vi "RS232 S&R 3.vi"(4 "ReSetSPD":bool, 5 "error in":errorcluster, 6 "Delay (ms)":u32, 7 "Stage Control":T1={"Task"=0, "Position to go"={"Position"={"X"=FALSE, "Target X (um)"=1000.0, "Current X (um)"=1000.0, "Scaling X"=0, "Y"=FALSE, "Target Y (um)"=0.0, "Current Y (um)"=0.0, "Scaling Y"=0, "Z"=FALSE, "Target Z (um)"=0.0, "Current Z (um)"=0.0, "Scaling Z"=0}, "Speed"={"Speed"=3111, "Vi steps"=800, "Vi"=1000}}} {"Task" items=["MOVE", "HOME", "STOP", "Set Speed", "Info", "Set Zero", "MOVE2"]; "Position to go"."Speed"."Speed" min=50 max=8000 step=50 scale=50.0..8000.0; "Position to go"."Position"."Current X (um)" step=1.0; "Position to go"."Position"."Scaling Z" items=["X", "Z", "None"]; "Position to go"."Position"."Scaling Y" items=["X", "Z", "None"]; "Position to go"."Position"."Scaling X" items=["X", "Z", "None"]; "Position to go"."Position"."Target X (um)" step=1.0}, 8 "VISA resource in":refnum<visa-resource-name>) -> (0 "error out":errorcluster, 1 "read":bool, 2 "Cluster":T2={"Current coordinates"={"Steps"=0.0, "X"=FALSE, "Steps 2"=0.0, "Y"=FALSE, "Steps 3"=0.0, "Z"=FALSE}, "read buffer"="X0,Y0,Z0\r\n", "Command"="a", "Current coordinates 2"={"X"=0.0, "Y"=0.0, "Z"=0.0}, "Moving Time (Sec)"=0.0}, 3 "VISA resource name out":refnum<visa-resource-name>)   [LabVIEW 2018]
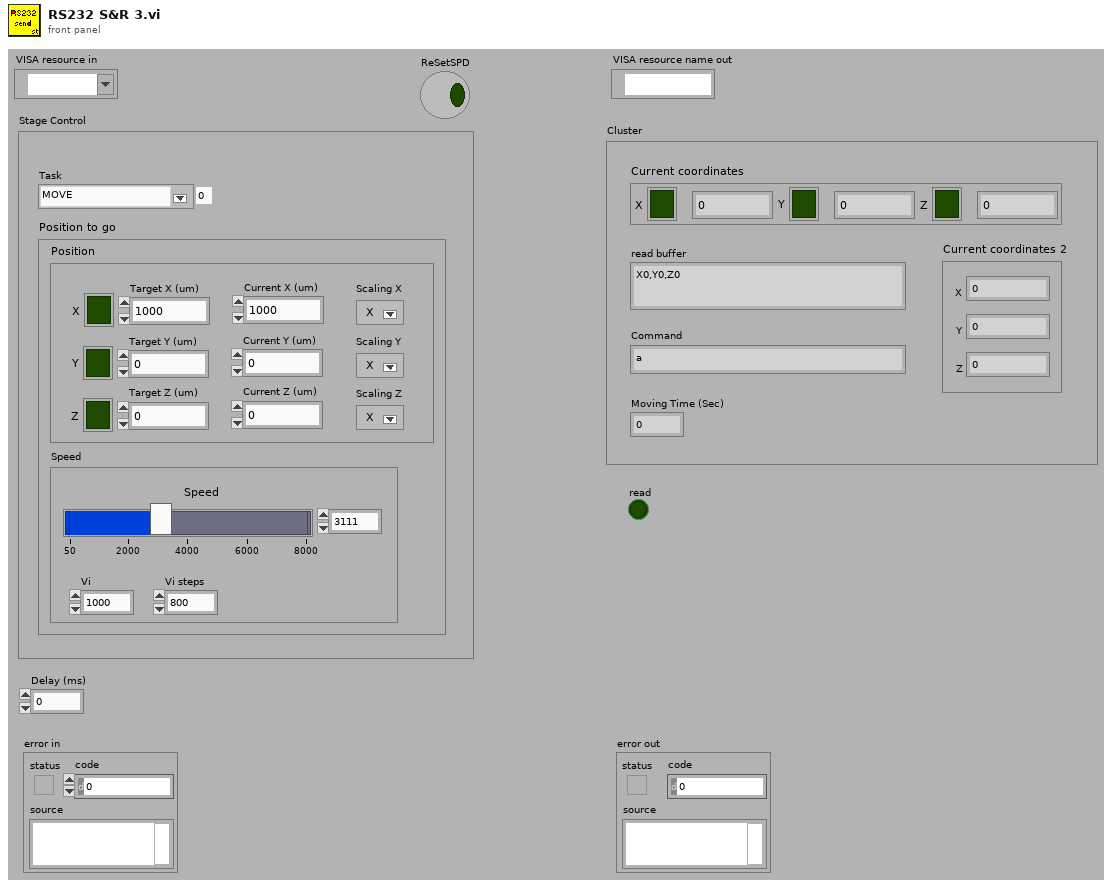
[diagram p1: front panel]
types:
  T1 = cluster{"Task":u16, "Position to go":cluster{"Position":cluster{"X":bool, "Target X (um)":dbl, "Current X (um)":dbl, "Scaling X":u16, "Y":bool, "Target Y (um)":dbl, "Current Y (um)":dbl, "Scaling Y":u16, "Z":bool, "Target Z (um)":dbl, "Current Z (um)":dbl, "Scaling Z":u16}, "Speed":cluster{"Speed":i32, "Vi steps":i32, "Vi":i32}}}
  T2 = cluster{"Current coordinates":cluster{"Steps":dbl, "X":bool, "Steps 2":dbl, "Y":bool, "Steps 3":dbl, "Z":bool}, "read buffer":string, "Command":string, "Current coordinates 2":cluster{"X":dbl, "Y":dbl, "Z":dbl}, "Moving Time (Sec)":dbl}
  T3 = cluster{"Position":cluster{"X":bool, "Target X (um)":dbl, "Current X (um)":dbl, "Scaling X":u16, "Y":bool, "Target Y (um)":dbl, "Current Y (um)":dbl, "Scaling Y":u16, "Z":bool, "Target Z (um)":dbl, "Current Z (um)":dbl, "Scaling Z":u16}, "Speed":cluster{"Speed":i32, "Vi steps":i32, "Vi":i32}}
  T4 = cluster{"X":bool, "Target X (um)":dbl, "Current X (um)":dbl, "Scaling X":u16, "Y":bool, "Target Y (um)":dbl, "Current Y (um)":dbl, "Scaling Y":u16, "Z":bool, "Target Z (um)":dbl, "Current Z (um)":dbl, "Scaling Z":u16}
  T5 = cluster{"X":bool, "Target X ":dbl, "Current X":dbl, "Scaling X":u16, "Y":bool, "Target Y":dbl, "Current Y":dbl, "Scaling Y":u16, "Z":bool, "Target Z":dbl, "Current Z":dbl, "Scaling Z":u16}
  T6 = cluster{"Steps":dbl, "X":bool, "Steps 2":dbl, "Y":bool, "Steps 3":dbl, "Z":bool}
  T7 = cluster{"Current coordinates":cluster{"Steps":dbl, "X":bool, "Steps 2":dbl, "Y":bool, "Steps 3":dbl, "Z":bool}, "read buffer":string, "command":string, cluster{"X":dbl, "Y":dbl, "Z":dbl}, dbl}
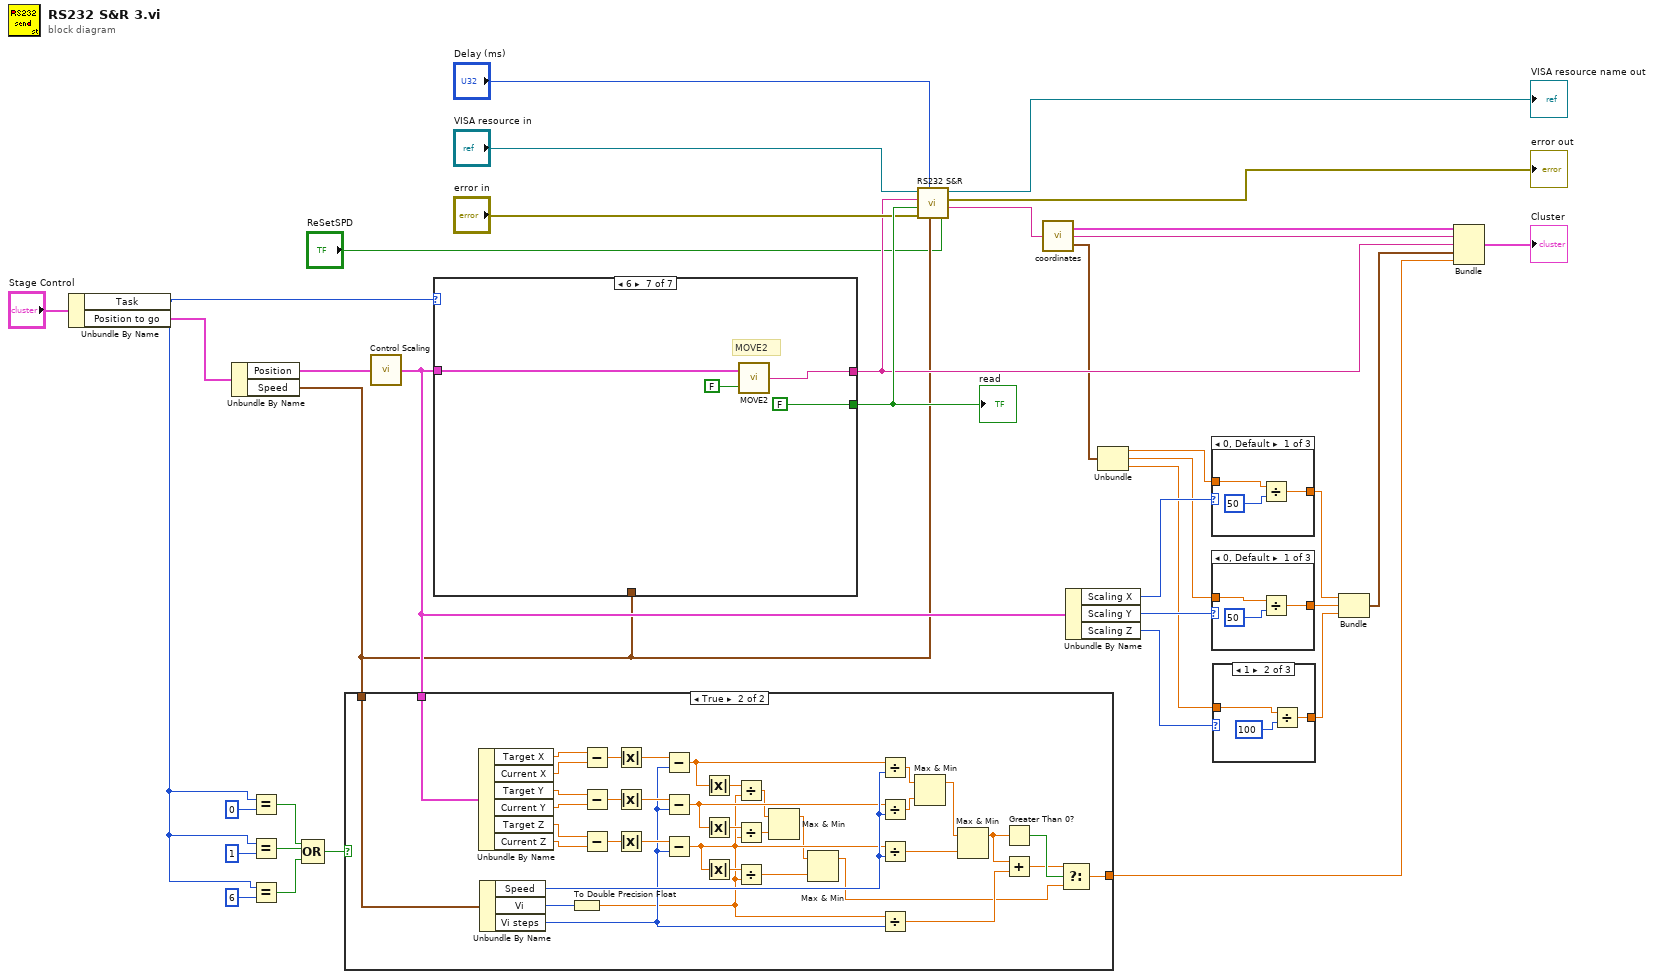
[diagram p0: block diagram]
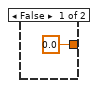
[diagram p2: hidden frame]
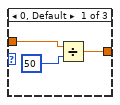
[diagram p3: hidden frame]
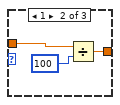
[diagram p5: hidden frame]
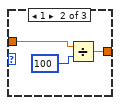
[diagram p7: hidden frame]
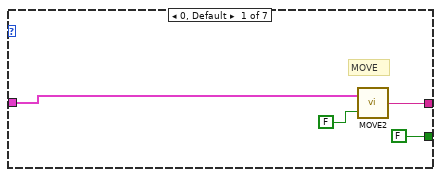
[diagram p9: hidden frame]
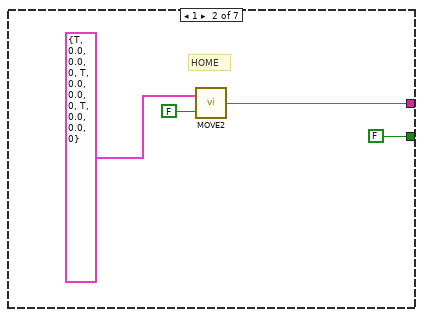
[diagram p10: hidden frame]
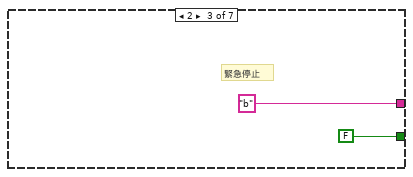
[diagram p11: hidden frame]
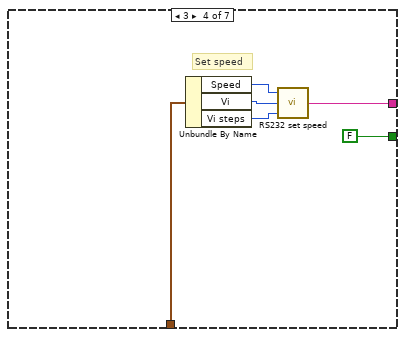
[diagram p12: hidden frame]
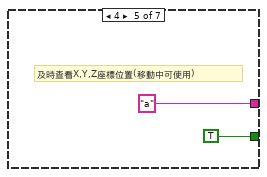
[diagram p13: hidden frame]
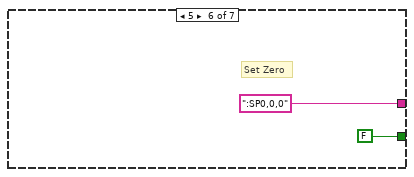
[diagram p14: hidden frame]
diagram:
  n1 = Unbundle By Name("Stage Control") -> ("Task"=w5:u16, "Position to go"=w10:T3)
  n2 = Unbundle By Name(w10) -> ("Position"=w13:T4, "Speed"=w12:cluster{"Speed":i32, "Vi steps":i32, "Vi":i32})
  n3 = Equal?(x=w5, y=u16 0) -> (x = y?=w4:bool)
  n4 = Equal?(x=w5, y=u16 1) -> (x = y?=w3:bool)
  n5 = Equal?(x=w5, y=u16 6) -> (x = y?=w2:bool)
  n6 = Compound Arithmetic op=OR(w4, w3, w2) -> (w1:bool)
  n7 = call "Control Scaling.vi"("Position to go"=w13) -> ("Position to go out"=w15:T5)
  n8 = case shown="True" w1 {
    tunnel: w15 -> [_ w75]
    tunnel: [0.0 w39] -> w14
    tunnel: w12 -> [_ w38]
    frame False {
    }
    frame True {
      n9 = Unbundle By Name(w75) -> ("Target X"=w73:dbl, "Current X"=w74:dbl, "Target Y"=w72:dbl, "Current Y"=w71:dbl, "Target Z"=w70:dbl, "Current Z"=w69:dbl)
      n10 = Unbundle By Name(w38) -> ("Speed"=w62:i32, "Vi"=w61:i32, "Vi steps"=w60:i32)
      n11 = To Double Precision Float(number=w61) -> (double precision float=w46:dbl)
      n12 = Subtract(x=w73, y=w74) -> (x-y=w68:dbl)
      n13 = Subtract(x=w72, y=w71) -> (x-y=w66:dbl)
      n14 = Subtract(x=w70, y=w69) -> (x-y=w67:dbl)
      n15 = Absolute Value(x=w68) -> (abs(x)=w65:dbl)
      n16 = Absolute Value(x=w66) -> (abs(x)=w64:dbl)
      n17 = Absolute Value(x=w67) -> (abs(x)=w63:dbl)
      n18 = Subtract(x=w65, y=w60) -> (x-y=w51:dbl)
      n19 = Subtract(x=w64, y=w60) -> (x-y=w47:dbl)
      n20 = Subtract(x=w63, y=w60) -> (x-y=w45:dbl)
      n21 = Absolute Value(x=w51) -> (abs(x)=w50:dbl)
      n22 = Absolute Value(x=w47) -> (abs(x)=w49:dbl)
      n23 = Absolute Value(x=w45) -> (abs(x)=w48:dbl)
      n24 = Divide(x=w50, y=w46) -> (x/y=w43:dbl)
      n25 = Divide(x=w49, y=w45) -> (x/y=w42:dbl)
      n26 = Divide(x=w48, y=w46) -> (x/y=w41:dbl)
      n27 = Max & Min(x=w43, y=w42) -> (max(x,y)=w44:dbl)  [unwired: 1 out]
      n28 = Max & Min(x=w44, y=w41) -> (max(x,y)=w40:dbl)  [unwired: 1 out]
      n29 = Divide(x=w51, y=w62) -> (x/y=w59:dbl)
      n30 = Divide(x=w47, y=w62) -> (x/y=w58:dbl)
      n31 = Divide(x=w45, y=w62) -> (x/y=w57:dbl)
      n32 = Divide(x=w46, y=w60) -> (x/y=w53:dbl)
      n33 = Max & Min(x=w59, y=w58) -> (max(x,y)=w56:dbl)  [unwired: 1 out]
      n34 = Max & Min(x=w56, y=w57) -> (max(x,y)=w54:dbl)  [unwired: 1 out]
      n35 = Greater Than 0?(x=w54) -> (x > 0?=w55:bool)
      n36 = Add(x=w54, y=w53) -> (x+y=w52:dbl)
      n37 = Select(t=w52, s=w55, f=w40) -> (s? t:f=w39:dbl)
    }
  }
  n38 = case shown="6" w5 {
    tunnel: [w79 w82 "b" ("Command") w87 "a" ":SP0,0,0" ("Command") w99] -> w29
    tunnel: [FALSE FALSE FALSE FALSE TRUE FALSE FALSE] -> w35
    tunnel: w15 -> [w76 _ _ _ _ _ w96]
    tunnel: w12 -> [_ _ _ w86 _ _ _]
    frame 0, Default {
      # "MOVE"
      n39 = call "MOVE2.vi"("Relative"=FALSE, "Position to go"=w76) -> ("command"=w79:string)
    }
    frame 1 {
      # "HOME"
      n40 = call "MOVE2.vi"("Relative"=FALSE, "Position to go"=T4 {"X"=TRUE, "Target X (um)"=0.0, "Current X (um)"=0.0, "Scaling X"=0, "Y"=TRUE, "Target Y (um)"=0.0, "Current Y (um)"=0.0, "Scaling Y"=0, "Z"=TRUE, "Target Z (um)"=0.0, "Current Z (um)"=0.0, "Scaling Z"=0}) -> ("command"=w82:string)
    }
    frame 2 {
      # "緊急停止"
    }
    frame 3 {
      # "Set speed"
      n41 = Unbundle By Name(w86) -> ("Speed"=w88:i32, "Vi"=w89:i32, "Vi steps"=w90:i32)
      n42 = call "RS232 set speed.vi"("Vi steps"=w90, "Vi"=w89, "Speed"=w88) -> ("Command"=w87:string)
    }
    frame 4 {
      # "及時查看X,Y,Z座標位置(移動中可使用)"
    }
    frame 5 {
      # "Set Zero"
    }
    frame 6 {
      # "MOVE2"
      n43 = call "MOVE2.vi"("Relative"=FALSE, "Position to go"=w96) -> ("command"=w99:string)
    }
  }
  "read" <- w35
  n44 = call "RS232 S&R.vi"("ReSetSP"="ReSetSPD", "Speed"=w12, "Delay (ms)"="Delay (ms)", "error in"="error in", "Read"=w35, "write buffer"=w29, "VISA resource in"="VISA resource in") -> ("read buffer"=w30:string, "error out"=→"error out":errorcluster, "VISA resource name out"=→"VISA resource name out":refnum<visa-resource-name>)
  n45 = call "coordinates.vi"("read buffer"=w30) -> (1:"Current coordinates"=w27:T6, 2:"Current coordinates"=w23:cluster{"X":dbl, "Y":dbl, "Z":dbl})
  n46 = Unbundle By Name(w15) -> ("Scaling X"=w26:u16, "Scaling Y"=w25:u16, "Scaling Z"=w24:u16)
  n47 = Unbundle(w23) -> ("X"=w22:dbl, "Y"=w21:dbl, "Z"=w20:dbl)
  n48 = case shown="0, Default" w26 {
    tunnel: w22 -> [w101 w104 w106]
    tunnel: [w100 w103 w106] -> w19
    frame 0, Default {
      n49 = Divide(x=w101, y=50) -> (x/y=w100:dbl)
    }
    frame 1 {
      n50 = Divide(x=w104, y=100) -> (x/y=w103:dbl)
    }
    frame 2 {
    }
  }
  n51 = case shown="0, Default" w25 {
    tunnel: w21 -> [w108 w111 w113]
    tunnel: [w107 w110 w113] -> w18
    frame 0, Default {
      n52 = Divide(x=w108, y=50) -> (x/y=w107:dbl)
    }
    frame 1 {
      n53 = Divide(x=w111, y=100) -> (x/y=w110:dbl)
    }
    frame 2 {
    }
  }
  n54 = case shown="1" w24 {
    tunnel: w20 -> [w115 w118 w120]
    tunnel: [w114 w117 w120] -> w17
    frame 0, Default {
      n55 = Divide(x=w115, y=50) -> (x/y=w114:dbl)
    }
    frame 1 {
      n56 = Divide(x=w118, y=100) -> (x/y=w117:dbl)
    }
    frame 2 {
    }
  }
  n57 = Bundle("X"=w19, "Y"=w18, "Z"=w17) -> (w16:cluster{"X":dbl, "Y":dbl, "Z":dbl})  [unwired: 1 in]
  n58 = Bundle("Current coordinates"=w27, "read buffer"=w30, "command"=w29, w16, w14) -> (→"Cluster":T7)  [unwired: 1 in]
